vi "Add Entity.vi"(7 "entity type":i32, 8 "error in (no error)":errorcluster, 9 "entity details":T1, 10 "enqueuer":refnum<class "Message Enqueuer.lvclass">, 11 "Entity Table in":refnum<class "Entity Table.lvclass">) -> (0 "error out":errorcluster, 3 "Entity Table out":refnum<class "Entity Table.lvclass">)   [LabVIEW 2023, in "Entity Table.lvclass"]
doc: "Add a new actor to the entity table."
uses:
  Entity Table.lvclass
  <vilib>/ActorFramework/Message Enqueuer/Message Enqueuer.lvclass
  Entity Data.ctl
  Entity Table.lvclass/Entity Table.ctl
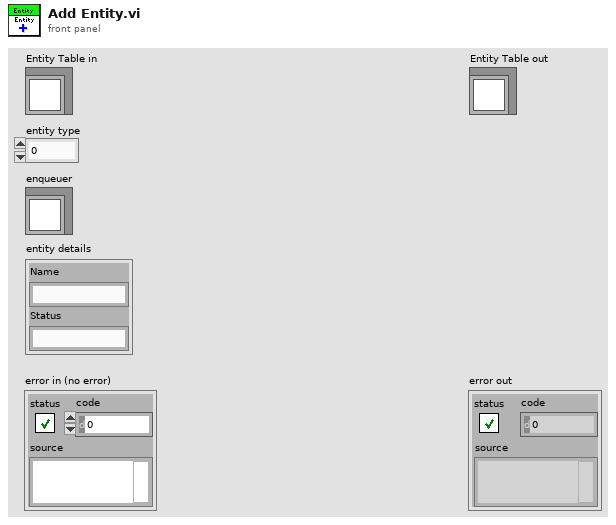
[diagram p1: front panel]
types:
  T1 = typedef "Entity Table.lvclass/Entity Data.ctl" = cluster{"Name":string, "Status":string}
  T2 = typedef "Entity Table.lvclass/Entity Table Element.ctl" = cluster{"Entity":refnum<class "Message Enqueuer.lvclass">[], "Entity Data":T1[]}
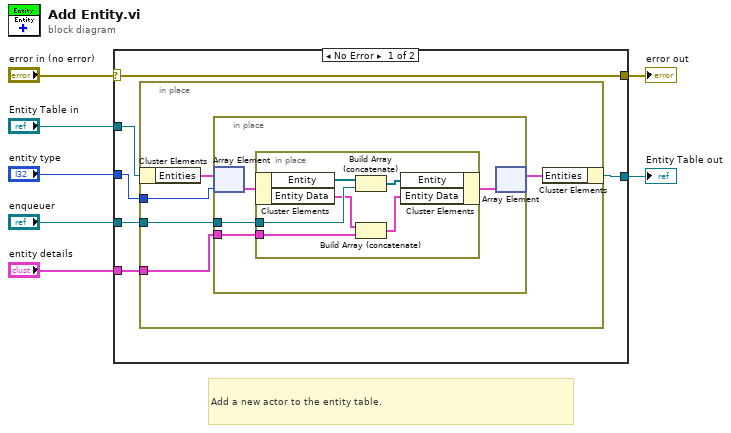
[diagram p0: block diagram]
diagram:
  # "Add a new actor to the entity table."
  n1 = case shown="No Error" "error in (no error)" {
    selector: "error in (no error)" -> [w11 w30]
    tunnel: [w11 w30] -> w6
    tunnel: "entity type" -> [w13 _]
    tunnel: "enqueuer" -> [w12 _]
    tunnel: "Entity Table in" -> [w9 w29]
    tunnel: [w8 w29] -> w1
    tunnel: "entity details" -> [w10 _]
    frame No Error {
      n2 = in-place "In Place Element Structure" {
        in-place-border: w13 -> [w18]
        in-place-border: w12 -> [w17]
        in-place-border: w10 -> [w16]
        n3 = in-place-cluster #1 ("Unbundle / Bundle Elements")(w9) -> ("Entities"=w15:T2[])
        n4 = in-place "In Place Element Structure" {
          in-place-border: w17 -> [w21]
          in-place-border: w16 -> [w19]
          n5 = in-place-array #2 ("Array Index / Replace Elements")(w15, w18) -> (w22:T2)
          n6 = in-place "In Place Element Structure" {
            in-place-border: w21 -> [w27]
            in-place-border: w19 -> [w24]
            n7 = in-place-cluster #3 ("Unbundle / Bundle Elements")(w22) -> ("Entity"=w28:refnum<class "Message Enqueuer.lvclass">[], "Entity Data"=w25:T1[])
            n8 = Build Array (concatenate)(w28, w27) -> (w26:refnum<class "Message Enqueuer.lvclass">[])
            n9 = Build Array (concatenate)(w25, w24) -> (w23:T1[])
            n10 = in-place-cluster #3 ("Unbundle / Bundle Elements")("Entity"=w26, "Entity Data"=w23) -> (w20:T2)
          }
          n11 = in-place-array #2 ("Array Index / Replace Elements")(w20) -> (w14:T2[])  [unwired: 1 out]
        }
        n12 = in-place-cluster #1 ("Unbundle / Bundle Elements")("Entities"=w14) -> (w8:refnum<class "Entity Table.lvclass">)
      }
    }
    frame Error {
    }
  }
  "error out" <- w6
  "Entity Table out" <- w1
